vi "Get Section Names.vi"(7 "Section Regex [\"\", all]":string, 8 "error in (no error)":errorcluster, 10 "Use Regex? [T]":bool=TRUE, 11 "Carya Config in":refnum<class "Carya Config.lvclass">) -> (0 "error out":errorcluster, 2 "Section names":string[](array[string]), 3 "Carya Config out":refnum<class "Carya Config.lvclass">)   [LabVIEW 2013, in "Carya Config.lvclass"]
doc: "Copyright 2018, Carya Automatisering, Wiebe Walstra."
uses:
  Carya Config.lvclass
  CConfig Object/Add Results Query/Add Results Query.lvclass
  CConfig Object/Loop Query/Match Query/Match Query.lvclass
  CConfig Object/Loop Query/All Query/All Query.lvclass
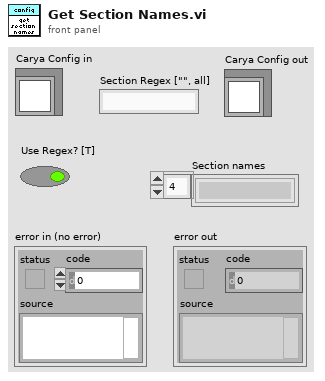
[diagram p1: front panel]
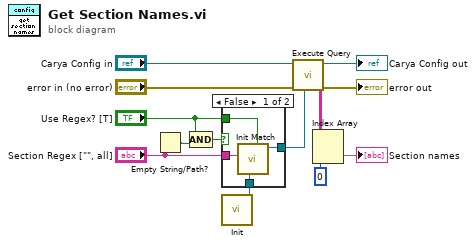
[diagram p0: block diagram]
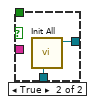
[diagram p2: hidden frame]
diagram:
  n1 = Empty String/Path?(string/path="Section Regex [\"\", all]") -> (empty?=w6:bool)
  n2 = Compound Arithmetic op=AND("Use Regex? [T]", w6) -> (w5:bool)
  n3 = call "Init.vi"() -> ("Find First Query out"=w2:refnum<class "Add Results Query.lvclass">)  [unwired: 10 in, 1 out]
  n4 = case shown="False" w5 {
    tunnel: "Use Regex? [T]" -> [w16 _]
    tunnel: "Section Regex [\"\", all]" -> [w17 _]
    tunnel: w2 -> [w15 w19]
    tunnel: [w14 w18] -> w1
    frame False {
      n5 = call "Init Match.vi"("Regex [F]"=w16, "Found"=w15, "Data"=w17) -> ("Find First Query out"=w14:refnum<class "Loop Query.lvclass">)  [unwired: 7 in, 1 out]
    }
    frame True {
      n6 = call "Init All.vi"("Found"=w19) -> ("Find First Query out"=w18:refnum<class "All Query.lvclass">)  [unwired: 9 in, 1 out]
    }
  }
  n7 = call-dynamic "Execute Query.vi"("Config Query in"=w1, "error in (no error)"="error in (no error)", "Carya Config in"="Carya Config in") -> ("error out"=→"error out":errorcluster, "Results"=w3:string[][], "Carya Config out"=→"Carya Config out":refnum<class "Carya Config.lvclass">)  [unwired: 4 in, 2 out]
  n8 = Index Array(array=w3, index (col)=0 ("disabled index (col)")) -> (element=→"Section names":string[])  [unwired: 1 in]
